vi "Teleop.vi"(10 "Match Info":T1={"Autonomous Elapsed Seconds"=0.0, "TeleOp Elapsed Seconds"=0.0, "Disabled Elapsed Seconds"=0.0, "Visited Autonomous"=FALSE, "Visited TeleOp"=FALSE, "Visited Disabled"=FALSE, "Autonomous Settings"={"Autonomous Style"=enum."Independent", "VI Refnum"=refnum}}, 11 "Call Context":T2) -> ()   [LabVIEW 2019]
doc: "This VI is called for each TeleOp packet received from the DS where the robot is not disabled. It is often used to read from the joysticks and update I/O or to update setpoints for timed control loops. It should complete and return within 20 milliseconds or it may miss DS packets."
uses:
  <vilib>/Rock Robotics/WPI/DriverStation/WPI_DriverStationDerivedRobotMode.ctl
  <vilib>/Rock Robotics/WPI/DriverStation/WPI_DriverStationMatch Info.ctl
  <vilib>/Rock Robotics/WPI/ThirdParty/Phoenix-LabVIEW/Motor Controller/Controls/CTRE_Phoenix_MotorControl_ControlMode.ctl
  <vilib>/Rock Robotics/Network Tables/NT Read Boolean.vi
  <vilib>/Rock Robotics/Network Tables/NT Read Number.vi
  <vilib>/Rock Robotics/WPI/Utilities/WPI_GetSetVariantRefNum.vi
  <vilib>/Rock Robotics/Network Tables/NT Write Numeric Array.vi
  <vilib>/Rock Robotics/Network Tables/NT Write Boolean Array.vi
  Robot Global Data.vi
panel:
  out "Shooter Stator Current":dbl
  out "Pulley Stator Current":dbl
  out "Kicket Stator Current":dbl
  out "Tank Drive Motor Values":dbl[](array[numeric])
  out "Sample Slider 0":dbl(slide) scale=0.0..5.0
  out "Sample Boolean 1":bool
  out "Sample Boolean 0":bool
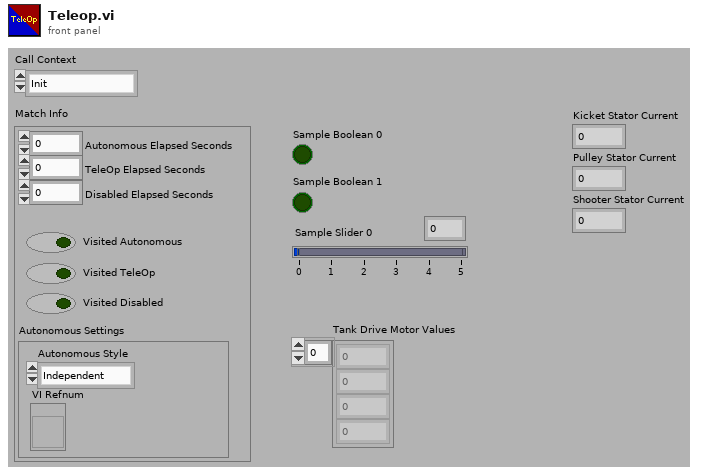
[diagram p1: front panel]
types:
  T1 = typedef "WPI_DriverStationMatch Info.ctl" = cluster{"Autonomous Elapsed Seconds":dbl, "TeleOp Elapsed Seconds":dbl, "Disabled Elapsed Seconds":dbl, "Visited Autonomous":bool, "Visited TeleOp":bool, "Visited Disabled":bool, "Autonomous Settings":cluster{"Autonomous Style":enum16{"Iterative", "Independent"}, "VI Refnum":refnum<vi>}}
  T2 = typedef "WPI_DriverStationDerivedRobotMode.ctl" = enum16{"Init", "Execute", "Stop"}
  T3 = typedef "CTRE_Phoenix_MotorControl_ControlMode.ctl" = u16
  T4 = typedef "WPI_JoystickDevRef.ctl" = cluster{"Device":T5}
  T5 = typedef "WPI_JoystickDeviceEnum.ctl" = enum16{"USB 0", "USB 1", "USB 2", "USB 3", "USB 4", "USB 5"}
  T6 = typedef "WPI_RobotDriveDevRef.ctl" = cluster{"DevStatus":errorcluster, "Motors[]":T7[], "Square Inputs":bool, "Max Output":dbl}
  T7 = typedef "WPI_MotorControlDeviceRef.ctl" = cluster{"DeviceStatus":errorcluster, "Type":T8, "PWM":cluster{"PWM Channel":T9, "DeadBand":T10}, "CAN":cluster{"Device Number":u8, "SetOutput VI Ref":variant, "GetOutput VI Ref":variant, "Enable VI Ref":variant, "Disable VI Ref":variant, "Data":variant}, "Invert":bool, "DIO PWM":cluster{"PWM \"Enable\" Channel":T9, "DIOChannel":T11, "PWM Rate":dbl}}
  T8 = typedef "WPI_MotorControlType.ctl" = enum16{"PWM", "CAN", "DIO PWM"}
  T9 = typedef "FPGA_DIOPWMChannel.ctl" = enum8{"PWM 0", "PWM 1", "PWM 2", "PWM 3", "PWM 4", "PWM 5", "PWM 6", "PWM 7", "PWM 8", "PWM 9", "PWM MXP 0", "PWM MXP 1", "PWM MXP 2", "PWM MXP 3", "PWM MXP 4", "PWM MXP 5", "PWM MXP 6", "PWM MXP 7", "PWM MXP 8", "PWM MXP 9", "Invalid"}
  T10 = typedef "WPI_PWMDeadband.ctl" = cluster{"Name":string, "maxPositivePwm":i32, "minPositivePwm":i32, "centerPwm":i32, "maxNegativePwm":i32, "minNegativePwm":i32, "angularRange":u16}
  T11 = typedef "FPGA_DIOChannel.ctl" = enum8{"DIO 0", "DIO 1", "DIO 2", "DIO 3", "DIO 4", "DIO 5", "DIO 6", "DIO 7", "DIO 8", "DIO 9", "DIO MXP 0", "DIO MXP 1", "DIO MXP 2", "DIO MXP 3", "DIO MXP 4", "DIO MXP 5", "DIO MXP 6", "DIO MXP 7", "DIO MXP 8", "DIO MXP 9", "DIO MXP 10", "DIO MXP 11", "DIO MXP 12", "DIO MXP 13", "DIO MXP 14", "DIO MXP 15", "SPI Port CS1", "SPI Port CS2", "SPI Port CS3", "SPI Port MISO", "SPI Port MOSI", "Invalid"}
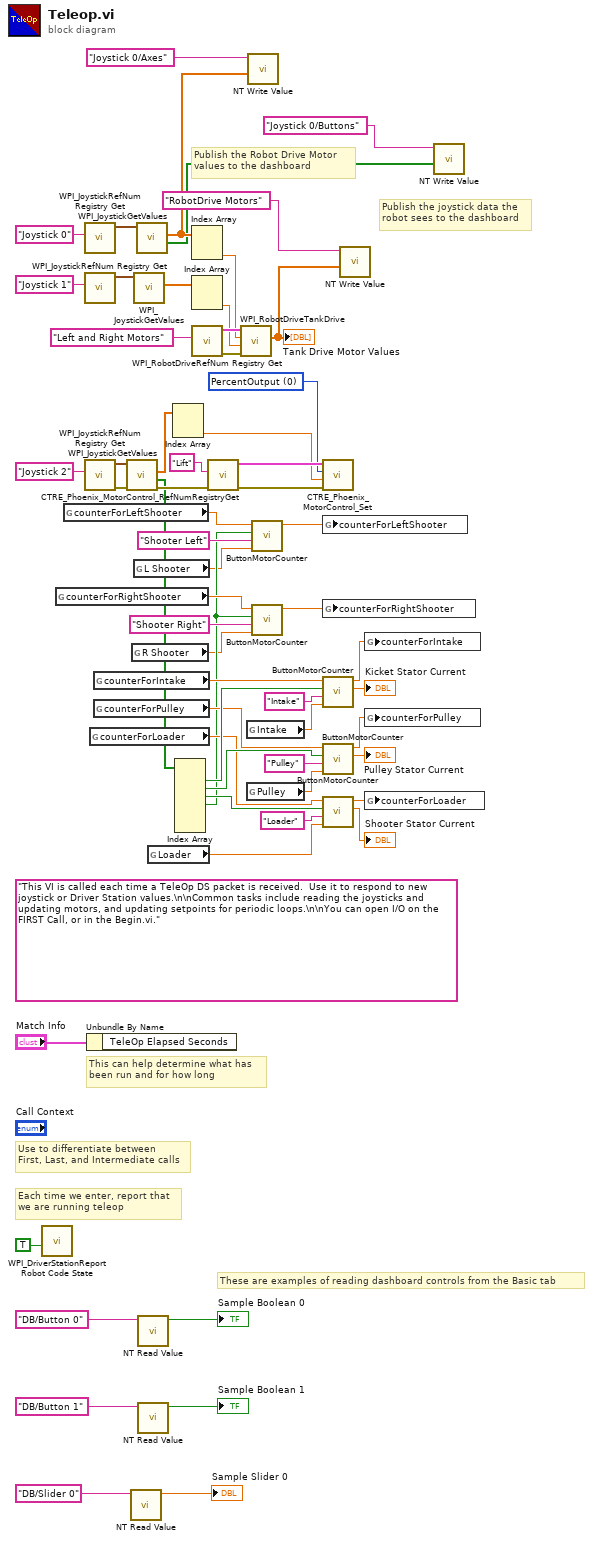
[diagram p0: block diagram]
diagram:
  w32 = T3 0 items=["PercentOutput"=0, "Position"=1, "Velocity"=2, "Current"=3, "Follower"=5, "MotionProfile"=6, "MotionMagic"=7, "MotionProfileArc"=10, "Disabled"=15] ("Control Mode")
  (unwired) "This VI is called each time a TeleOp DS packet is received.  Use it to respond to new joystick or Driver Station values.\n\nCommon tasks include reading the joysticks and updating motors, and updating setpoints for periodic loops.\n\nYou can open I/O on the FIRST Call, or in the Begin.vi."
  # "These are examples of reading dashboard controls from the Basic tab"
  # "Publish the Robot Drive Motor\nvalues to the dashboard"
  # "Publish the joystick data the\nrobot sees to the dashboard"
  # "Each time we enter, report that\nwe are running teleop"
  # "Use to differentiate between\nFirst, Last, and Intermediate calls"
  # "This can help determine what has\nbeen run and for how long"
  n1 = call <vilib>:"WPI_DriverStationReport Robot Code State.vi"("TeleOp"=TRUE ("Autonomous")) -> ()  [unwired: 10 in, 1 out]
  n2 = global read "Robot Global Data.vi" "counterForRightShooter"() -> (w7:dbl)
  n3 = global read "Robot Global Data.vi" "counterForLeftShooter"() -> (w10:dbl)
  n4 = call <vilib>:"WPI_JoystickRefNum Registry Get.vi"("refnum name"="Joystick 0") -> ("JoystickDevRef"=w47:T4)  [unwired: 1 in, 9 out]
  n5 = call <vilib>:"WPI_JoystickRefNum Registry Get.vi"("refnum name"="Joystick 1") -> ("JoystickDevRef"=w45:T4)  [unwired: 1 in, 9 out]
  n6 = call <vilib>:"WPI_JoystickRefNum Registry Get.vi"("refnum name"="Joystick 2") -> ("error out"=w35:errorcluster, "JoystickDevRef"=w37:T4)  [unwired: 1 in, 8 out]
  n7 = Unbundle By Name("Match Info") -> ()  [unwired: 1 out]
  n8 = global read "Robot Global Data.vi" "counterForLoader"() -> (w20:dbl)
  n9 = global read "Robot Global Data.vi" "counterForIntake"() -> (w24:dbl)
  n10 = global read "Robot Global Data.vi" "counterForPulley"() -> (w21:dbl)
  n11 = call <vilib>:"WPI_JoystickGetValues.vi"("error in (no error)"=w35, "JoystickDevRef"=w37) -> ("error out"=w30:errorcluster, "Buttons"=w28:bool[], "Axes"=w36:dbl[])  [unwired: 5 in, 2 out]
  n12 = call-poly <vilib>:"NT Read Value.vi"("Name"="DB/Slider 0" ("refnum name")) -> ("Numeric"=→"Sample Slider 0":dbl)  [unwired: 9 in, 1 out]
  n13 = global read "Robot Global Data.vi" "R Shooter"() -> (w5:dbl)
  n14 = call <vilib>:"WPI_JoystickGetValues.vi"("JoystickDevRef"=w45) -> ("Axes"=w44:dbl[])  [unwired: 6 in, 4 out]
  n15 = global read "Robot Global Data.vi" "L Shooter"() -> (w3:dbl)
  n16 = call <vilib>:"WPI_JoystickGetValues.vi"("JoystickDevRef"=w47) -> ("Buttons"=w39:bool[], "Axes"=w40:dbl[])  [unwired: 6 in, 3 out]
  n17 = call-poly <vilib>:"NT Read Value.vi"("Name"="DB/Button 0" ("refnum name")) -> ("Boolean"=→"Sample Boolean 0":bool)  [unwired: 9 in, 1 out]
  n18 = call-poly <vilib>:"NT Read Value.vi"("Name"="DB/Button 1" ("refnum name")) -> ("Boolean"=→"Sample Boolean 1":bool)  [unwired: 9 in, 1 out]
  n19 = global read "Robot Global Data.vi" "Loader"() -> (w1:dbl)
  n20 = Index Array(array=w36) -> (element #2=w31:dbl)  [unwired: 2 in, 1 out]
  n21 = Index Array(array=w28) -> (element #1=w27:bool, element #2=w23:bool, element #3=w22:bool, element #4=w6:bool)  [unwired: 7 in, 3 out]
  n22 = Index Array(array=w40) -> (element #2=w43:dbl)  [unwired: 2 in, 1 out]
  n23 = Index Array(array=w44) -> (element #2=w42:dbl)  [unwired: 2 in, 1 out]
  n24 = call <vilib>:"WPI_RobotDriveRefNum Registry Get.vi"("refnum name"="Left and Right Motors") -> ("error out"=w49:errorcluster, "RobotDriveDevRef"=w50:T6)  [unwired: 9 in]
  n25 = call <vilib>:"CTRE_Phoenix_MotorControl_RefNumRegistryGet.vi"("error in (no error)"=w30, "refnum name"="Lift") -> ("error out"=w29:errorcluster, "PhoenixMotorControlDevRef"=w33:T7)  [unwired: 8 in]
  n26 = call <vilib>:"WPI_RobotDriveTankDrive.vi"("error in (no error)"=w49, "Right axis value"=w42, "Left axis value"=w43, "RobotDriveDevRef"=w50) -> ("Motor Values"=w41:dbl[])  [unwired: 5 in, 2 out]
  "Tank Drive Motor Values" <- w41
  n27 = global read "Robot Global Data.vi" "Intake"() -> (w4:dbl)
  n28 = global read "Robot Global Data.vi" "Pulley"() -> (w2:dbl)
  n29 = call-poly <vilib>:"NT Write Value.vi"("Numeric Array"=w40, "Name"="Joystick 0/Axes") -> ()  [unwired: 9 in, 1 out]
  n30 = call "ButtonMotorCounter.vi"("Motor Set Point"=w3, "refnum name"="Shooter Left", "Boolean"=w6, "counterForIntake in"=w10) -> ("counterForIntake out"=w12:dbl)  [unwired: 6 in, 1 out]
  n31 = call "ButtonMotorCounter.vi"("Motor Set Point"=w5, "refnum name"="Shooter Right", "Boolean"=w6, "counterForIntake in"=w7) -> ("counterForIntake out"=w9:dbl)  [unwired: 6 in, 1 out]
  n32 = call <vilib>:"CTRE_Phoenix_MotorControl_Set.vi"("error in (no error)"=w29, "Output"=w31, "Control Mode"=w32, "PhoenixMotorControlDevRef"=w33) -> ()  [unwired: 6 in, 2 out]
  n33 = global write "Robot Global Data.vi" "counterForLeftShooter"(w12) -> ()
  n34 = global write "Robot Global Data.vi" "counterForRightShooter"(w9) -> ()
  n35 = call "ButtonMotorCounter.vi"("Motor Set Point"=w4, "refnum name"="Intake", "Boolean"=w27, "counterForIntake in"=w24) -> ("Stator Current"=→"Kicket Stator Current":dbl, "counterForIntake out"=w26:dbl)  [unwired: 6 in]
  n36 = call "ButtonMotorCounter.vi"("Motor Set Point"=w2, "refnum name"="Pulley", "Boolean"=w23, "counterForIntake in"=w21) -> ("Stator Current"=→"Pulley Stator Current":dbl, "counterForIntake out"=w19:dbl)  [unwired: 6 in]
  n37 = call "ButtonMotorCounter.vi"("Motor Set Point"=w1, "refnum name"="Loader", "Boolean"=w22, "counterForIntake in"=w20) -> ("Stator Current"=→"Shooter Stator Current":dbl, "counterForIntake out"=w18:dbl)  [unwired: 6 in]
  n38 = call-poly <vilib>:"NT Write Value.vi"("Numeric Array"=w41, "Name"="RobotDrive Motors") -> ()  [unwired: 9 in, 1 out]
  n39 = global write "Robot Global Data.vi" "counterForIntake"(w26) -> ()
  n40 = global write "Robot Global Data.vi" "counterForPulley"(w19) -> ()
  n41 = global write "Robot Global Data.vi" "counterForLoader"(w18) -> ()
  n42 = call-poly <vilib>:"NT Write Value.vi"("Boolean Array"=w39, "Name"="Joystick 0/Buttons") -> ()  [unwired: 9 in, 1 out]
